vi "Fast IV Contour_VoltageField_outdate.vi"(8 "error in":errorcluster, 11 "Book number":i32=147) -> (0 "error out":errorcluster)   [LabVIEW 2017]
uses:
  <vilib>/Utility/file.llb/Write Delimited Spreadsheet (DBL).vi
  global.vi
panel:
  in  "Agi Address":refnum<visa-resource-name>="GPIB0::10::INSTR"
  in  "SRS resource name":refnum<visa-resource-name>="GPIB0::19::INSTR"
  in  "Agi T or SRS F":bool=TRUE
  in  "Ramp Rate V per Sec":dbl=0.04
  in  "Field Output Channel":i32=1
  in  "Field-DAQ Device Number":i32=1
  in  "Field Readout":tag="Dev1/ai3"
  in  "Average times":i32=30
  in  "Current step uA":dbl=0.007 format="%#_13g"
  in  "Voltage Read  channel":tag="Dev1/ai1"
  in  "samples per channel":i32=2000
  in  "Trigger source":tag="/Dev1/PFI12"
  in  "DAQ rate":dbl=100000.0 format="%#_13g"
  in  "Scale factor":dbl=1.0
  out "Current Field mT":dbl=-1.172
  in  "Frequency Hz":dbl=50.0
  in  "Vmax":dbl=7.0
  out "Current Field V":dbl=-1.172
  in  "Contour plot folder":path=path "\\\\ad.uillinois.edu\\engr/mrl-dvh-research/Guang Yue/data/Contour plot"
  in  "End field V":dbl=2.0 format="%#_13g"
  in  "Field step V":dbl=0.004 format="%#_13g"
  in  "Start field V":dbl=-2.0 format="%#_13g"
  # "Check DAQ fast IV.vi to set default values ex scale factor etc."
  # "V_Field*Scale=mT"
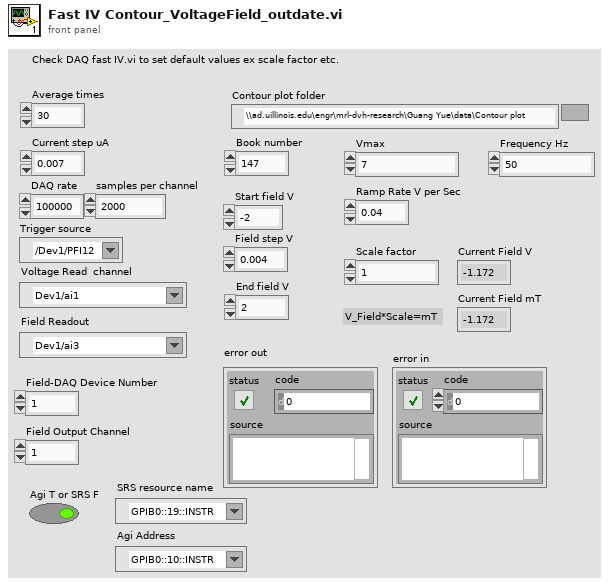
[diagram p1: front panel]
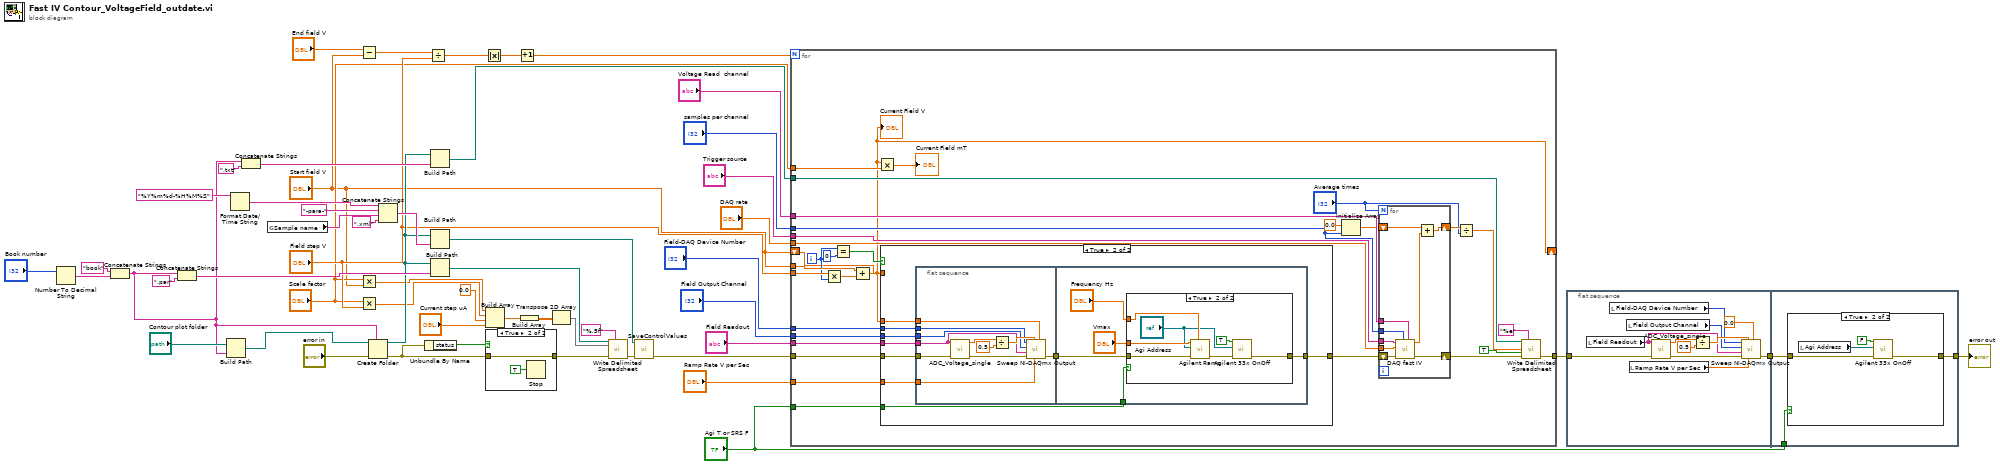
[diagram p0: block diagram]
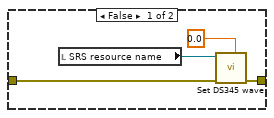
[diagram p2: hidden frame]
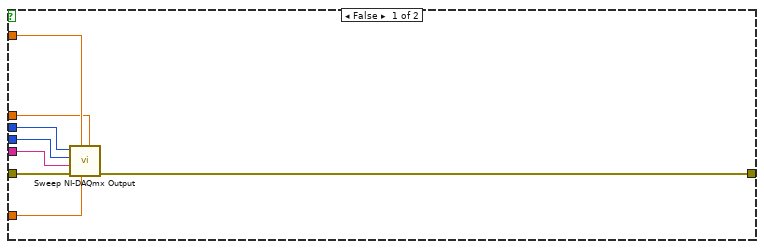
[diagram p4: hidden frame]
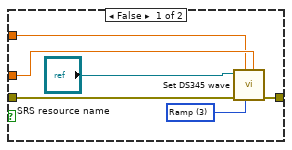
[diagram p5: hidden frame]
diagram:
  n1 = Number To Decimal String(number="Book number") -> (decimal integer string=w4:string)  [unwired: 1 in]
  n2 = Concatenate Strings("book" ("string"), w4) -> (w2:string)
  n3 = Concatenate Strings(w2, ".par" ("string")) -> (w42:string)
  n4 = Build Path(base path="Contour plot folder", name or relative path=w2) -> (appended path=w32:path)
  n5 = Format Date/Time String(time format string (%c)="%Y%m%d-%H%M%S") -> (date/time string=w26:string)  [unwired: 2 in]
  n6 = Concatenate Strings(w2, ".txt" ("string")) -> (w35:string)
  n7 = global read "global.vi" "Sample name"() -> (w25:string)
  n8 = Subtract(x="End field V", y="Start field V") -> (x-y=w53:dbl)
  n9 = Multiply(x="Scale factor", y="Start field V") -> (x*y=w16:dbl)
  n10 = Multiply(x="Scale factor", y="Field step V") -> (x*y=w13:dbl)
  n11 = Create Folder(prompt (Create Folder)=w2, path (use dialog)=w32, error in="error in") -> (created path=w27:path, error out=w29:errorcluster)  [unwired: 1 out]
  n12 = Concatenate Strings(w26, "-para-" ("string"), w25, ".xml" ("string")) -> (w46:string)
  n13 = Unbundle By Name(w29) -> ("status"=w30:bool)
  n14 = Divide(x=w53, y="Field step V") -> (x/y=w52:dbl)
  n15 = Build Path(base path=w27, name or relative path=w35) -> (appended path=w34:path)
  n16 = Build Path(base path=w27, name or relative path=w46) -> (appended path=w44:path)
  n17 = Build Path(base path=w27, name or relative path=w42) -> (appended path=w41:path)
  n18 = Absolute Value(x=w52) -> (abs(x)=w51:dbl)
  n19 = Build Array(w16, w13, 0.0 ("element"), "Current step uA") -> (w39:dbl[])
  n20 = case shown="True" w30 {
    tunnel: [w55 w57] -> w28
    tunnel: w29 -> [w55 w57]
    frame False {
    }
    frame True {
      n21 = Stop(stop? (T)=TRUE) -> ()
    }
  }
  n22 = Increment(x=w51) -> (x+1=w50:dbl)
  n23 = Build Array(w39) -> (w38:dbl[][])
  n24 = Transpose 2D Array(2D array=w38) -> (transposed array=w37:dbl[][])
  n25 = call-poly <vilib>:"Write Delimited Spreadsheet.vi"("file path (dialog if empty)"=w41, "format (%.3f)"="%.5f", "2D data"=w37, "error in (no error)"=w28) -> ("error out"=w31:errorcluster)  [unwired: 10 in, 1 out]
  n26 = call "SaveControlValues.vi"("XML File Path"=w44, "error in (no error)"=w31) -> ("error out"=w24:errorcluster)  [unwired: 8 in]
  n27 = for {
    N: w50 -> [_]
    tunnel: "Start field V" -> [w87]
    tunnel: "Field step V" -> [w86]
    tunnel: w34 -> [w81]
    tunnel: w24 -> [w79]
    tunnel: [w76] -> w23
    tunnel: "Voltage Read  channel" -> [w74]
    tunnel: "samples per channel" -> [w66]
    tunnel: "Trigger source" -> [w73]
    tunnel: "DAQ rate" -> [w72]
    tunnel: "Scale factor" -> [w71]
    tunnel: "Field Readout" -> [w64]
    tunnel: "Field-DAQ Device Number" -> [w63]
    tunnel: "Field Output Channel" -> [w62]
    tunnel: "Ramp Rate V per Sec" -> [w61]
    shift-right: [w60] -> _
    shift-left: "Start field V" -> [w59]
    tunnel: "Agi T or SRS F" -> [w58]
    i -> [w85]
    n28 = Multiply(x=w86, y=w85) -> (x*y=w88:dbl)
    n29 = Equal?(x=w85, y=0) -> (x = y?=w80:bool)
    n30 = Add(x=w87, y=w88) -> (x+y=w60:dbl)
    "Current Field V" <- w60
    n31 = Multiply(x=w60, y=w71) -> (x*y=→"Current Field mT":dbl)
    n32 = case shown="True" w80 {
      tunnel: w79 -> [w102 w113]
      tunnel: [w101 w112] -> w78
      tunnel: w60 -> [w99 w114]
      tunnel: w64 -> [w103 w111]
      tunnel: w63 -> [w105 w109]
      tunnel: w62 -> [w104 w108]
      tunnel: w61 -> [w98 w107]
      tunnel: w59 -> [w100 _]
      tunnel: w58 -> [_ w106]
      frame False {
        n33 = call "Sweep NI-DAQmx Output.vi"("Final Output Value"=w99, "Ramp Rate V/s"=w98, "Init Input Voltage"=w100, "error in"=w102, "Field Read Voltage"=w103, "Output Channel"=w104, "NI-DAQ Device Number"=w105) -> ("error out"=w101:errorcluster)  [unwired: 4 in]
      }
      frame True {
        n34 = flat-sequence {
          tunnel: w114 -> [w116]
          tunnel: w113 -> [w121]
          tunnel: w111 -> [w117]
          tunnel: [w120] -> w110
          tunnel: w109 -> [w119]
          tunnel: w108 -> [w118]
          tunnel: w107 -> [w115]
          tunnel: [w130] -> w112
          tunnel: w110 -> [w127]
          tunnel: w106 -> [w126]
          frame #0 {
            n35 = call "ADC_Voltage_single.vi"("error in"=w121, "physical channels"=w117) -> ("error out"=w125:errorcluster, "data"=w124:dbl)  [unwired: 8 in]
            n36 = Divide(x=w124, y=0.5) -> (x/y=w122:dbl)
            n37 = call "Sweep NI-DAQmx Output.vi"("Final Output Value"=w116, "Ramp Rate V/s"=w115, "Init Input Voltage"=w122, "error in"=w125, "Field Read Voltage"=w117, "Output Channel"=w118, "NI-DAQ Device Number"=w119) -> ("error out"=w120:errorcluster)  [unwired: 4 in]
          }
          frame #1 {
            n38 = case shown="True" w126 {
              tunnel: [w133 w142] -> w130
              tunnel: "Vmax" -> [w132 w140]
              tunnel: "Frequency Hz" -> [w131 w139]
              tunnel: w127 -> [w134 w138]
              frame False {
                w136 = u16 3 items=["Sine", "Square", "Triangle", "Ramp", "Noise"] ("Waveform Function (0: Sine)")
                n39 = call "Set DS345 wave.vi"("Amplitude (0.01 Vpp)"=w132, "Waveform Function (0: Sine)"=w136, "Frequency (1000 Hz)"=w131, "error in (no error)"=w134, "VISA resource name"="SRS resource name") -> ("error out"=w133:errorcluster)  [unwired: 6 in]
              }
              frame True {
                n40 = call "Agilent Ramp.vi"("Frequency Hz"=w139, "error in (no error)"=w138, "VISA resource name"="Agi Address", "Vmax"=w140) -> ("error out"=w143:errorcluster)  [unwired: 7 in]
                n41 = call "Agilent 33x OnOff.vi"("error in (no error)"=w143, "VISA resource name"="Agi Address", "Enable Output  (T: Enable)"=TRUE) -> ("error out"=w142:errorcluster)  [unwired: 8 in]
              }
            }
          }
        }
      }
    }
    n42 = Initialize Array(0.0 ("element"), w66) -> (w65:dbl[])
    n43 = for {
      N: "Average times" -> [_]
      tunnel: w74 -> [w95]
      tunnel: w66 -> [w94]
      tunnel: w73 -> [w93]
      tunnel: w72 -> [w92]
      shift-right: [w96] -> w77
      shift-left: w78 -> [w97]
      shift-right: [w90] -> w70
      shift-left: w65 -> [w89]
      n44 = call "DAQ fast IV.vi"("physical channels"=w95, "samples per channel"=w94, "error in"=w97, "rate"=w92, "Trigger source"=w93) -> ("error out"=w96:errorcluster, "data"=w91:dbl[])  [unwired: 5 in]
      n45 = Add(x=w89, y=w91) -> (x+y=w90:dbl[])
    }
    n46 = Divide(x=w70, y="Average times") -> (x/y=w68:dbl[])
    n47 = call-poly <vilib>:"Write Delimited Spreadsheet.vi"("file path (dialog if empty)"=w81, "format (%.3f)"="%e", "1D data"=w68, "append to file? (new file:F)"=TRUE ("append to file? (F)"), "error in (no error)"=w77) -> ("error out"=w76:errorcluster)  [unwired: 9 in, 1 out]
  }
  n48 = flat-sequence {
    tunnel: w23 -> [w149]
    tunnel: [w148] -> w21
    tunnel: [w156] -> w22
    tunnel: w21 -> [w157]
    tunnel: "Agi T or SRS F" -> [w155]
    frame #0 {
      n49 = local read "Field Readout"() -> (w147:tag)
      n50 = local read "Field-DAQ Device Number"() -> (w146:i32)
      n51 = local read "Field Output Channel"() -> (w145:i32)
      n52 = local read "Ramp Rate V per Sec"() -> (w144:dbl)
      n53 = call "ADC_Voltage_single.vi"("error in"=w149, "physical channels"=w147) -> ("error out"=w154:errorcluster, "data"=w153:dbl)  [unwired: 8 in]
      n54 = Divide(x=w153, y=0.5) -> (x/y=w151:dbl)
      n55 = call "Sweep NI-DAQmx Output.vi"("Final Output Value"=0.0, "Ramp Rate V/s"=w144, "Init Input Voltage"=w151, "error in"=w154, "Field Read Voltage"=w147, "Output Channel"=w145, "NI-DAQ Device Number"=w146) -> ("error out"=w148:errorcluster)  [unwired: 4 in]
    }
    frame #1 {
      n56 = case shown="True" w155 {
        tunnel: w157 -> [w161 w165]
        tunnel: [w160 w164] -> w156
        frame False {
          n57 = local read "SRS resource name"() -> (w158:refnum<visa-resource-name>)
          n58 = call "Set DS345 wave.vi"("Amplitude (0.01 Vpp)"=0.0, "error in (no error)"=w161, "VISA resource name"=w158) -> ("error out"=w160:errorcluster)  [unwired: 8 in]
        }
        frame True {
          n59 = local read "Agi Address"() -> (w162:refnum<visa-resource-name>)
          n60 = call "Agilent 33x OnOff.vi"("error in (no error)"=w165, "VISA resource name"=w162, "Enable Output  (T: Enable)"=FALSE) -> ("error out"=w164:errorcluster)  [unwired: 8 in]
        }
      }
    }
  }
  "error out" <- w22
